vi "TCP Server Lookup Connection Info by Instance VI.vi"(8 "error in (no error)":errorcluster, 10 "Instance VI Refnum":refnum<vi>, 11 "TCP Server":refnum<class "JKI TCP Server.lvclass">) -> (0 "error out":errorcluster, 1 "OK to Start New Handler?":bool, 2 "Connection Info":T2, 3 "TCP Server out":refnum<class "JKI TCP Server.lvclass">, 4 "Additional Data":variant, 5 "Handler VI RefNum":T1)   [LabVIEW 2020, in "JKI TCP Server.lvclass"]
uses:
  JKI TCP Server.lvclass
  _Data Structures/TCP Server Connection Info Cluster.ctl
  _Data Structures/TCP Server Handler RefNum.ctl
  JKI TCP Server.lvclass/JKI TCP Server.ctl
panel:
  # "Copyright © 2004-2008 JKI. All rights reserved.\n\nAuthor: Jim Kring [jim.kring@jameskring.com]\n\nThis library is provided \"AS IS\" ,WITHOUT WARRANTIES OR \nCONDITIONS OF ANY KIND, either express or implied.\n\nJames Kring, Inc. -- http://www.jameskring.com"
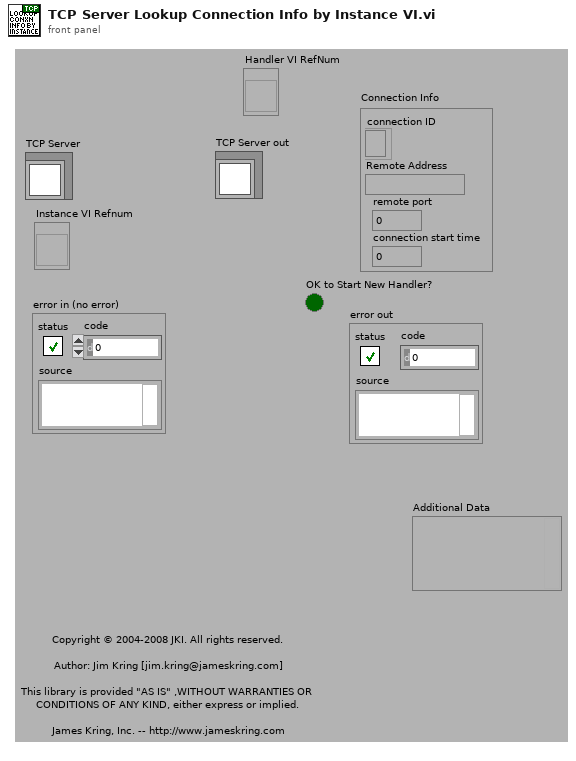
[diagram p1: front panel]
types:
  T1 = typedef "JKI TCP Server.lvclass/TCP Server Handler RefNum.ctl" = refnum<vi>
  T2 = typedef "JKI TCP Server.lvclass/TCP Server Connection Info Cluster.ctl" = cluster{"connection ID":refnum<k5>, "Remote Address":string, "remote port":u16, "connection start time":u32}
  T3 = typedef "JKI TCP Server.lvclass/TCP Server Data.ctl" = cluster{"Listener Info":T4, "Connection Process VI RefNums":refnum<vi>[], "dup connection IDs (for quick search)":refnum<k5>[], "Connections":T2[], "Connection Handler VI Path":path, "Handler Is Reentrant?":bool, "TCP Handler Instance RefNums":T1[], "TCP Handler VI RefNum":T1, "No. Connections":u32, "Max Connections":u32, "server start time":u32, "Additional Data":variant}
  T4 = typedef "JKI TCP Server.lvclass/TCP Server Listener Info Cluster.ctl" = cluster{"listener ID":refnum<k5>, "net address":u32, "port":u16, "Listener Process VI Refnum":refnum<vi>}
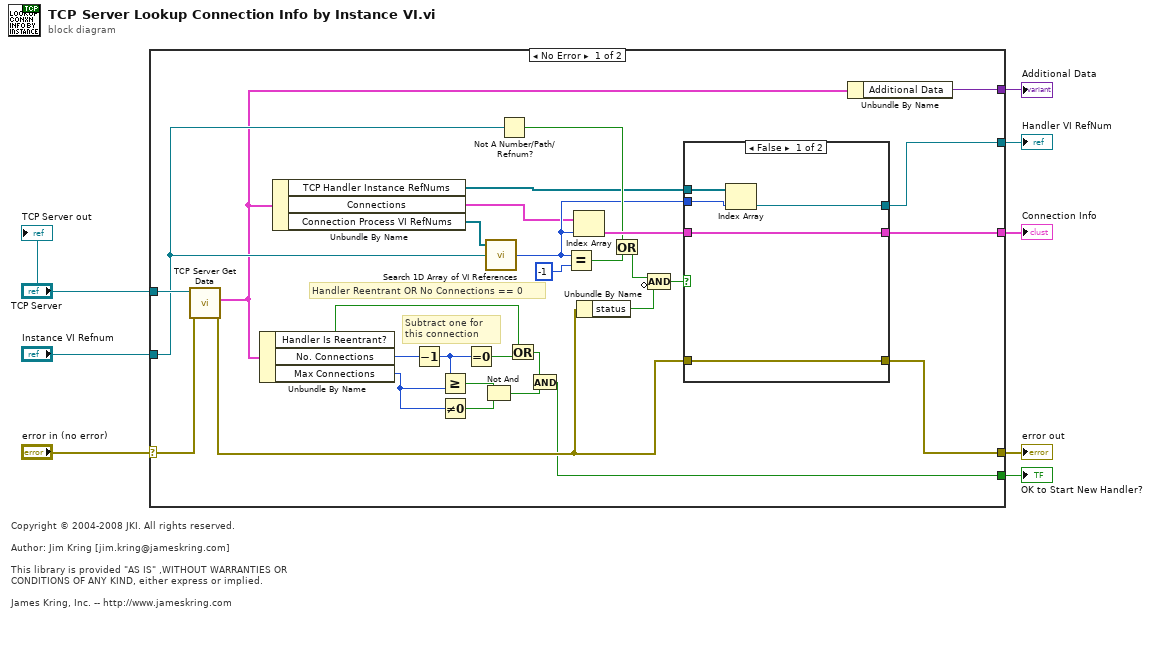
[diagram p0: block diagram]
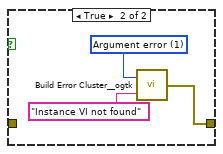
[diagram p2: hidden frame]
diagram:
  # "Copyright © 2004-2008 JKI. All rights reserved.\n\nAuthor: Jim Kring [jim.kring@jameskring.com]\n\nThis library is provided \"AS IS\" ,WITHOUT WARRANTIES OR \nCONDITIONS OF ANY KIND, either express or implied.\n\nJames Kring, Inc. -- http://www.jameskring.com"
  n1 = case shown="No Error" "error in (no error)" {
    tunnel: "TCP Server" -> [w38 _]
    tunnel: "Instance VI Refnum" -> [w27 _]
    tunnel: [w29 w47] -> w7
    selector: "error in (no error)" -> [w36 w47]
    tunnel: [w31 _] -> w4
    tunnel: [w22 _] -> w3
    tunnel: [w13 _] -> w2
    tunnel: [w10 _] -> w1
    frame No Error {
      # "Subtract one for this connection"
      # "Handler Reentrant OR No Connections == 0"
      n2 = call "TCP Server Get Data.vi"("error in (no error)"=w36, "TCP Server"=w38) -> ("error out"=w30:errorcluster, "Data out"=w11:T3)  [unwired: 7 in, 1 out]
      n3 = Unbundle By Name(w11) -> ("Handler Is Reentrant?"=w21:bool, "No. Connections"=w19:u32, "Max Connections"=w18:u32)
      n4 = Unbundle By Name(w11) -> ("TCP Handler Instance RefNums"=w24:T1[], "Connections"=w9:T2[], "Connection Process VI RefNums"=w37:refnum<vi>[])
      n5 = Decrement(x=w19) -> (x-1=w12:u32)
      n6 = Greater Or Equal?(x=w12, y=w18) -> (x >= y?=w17:bool)
      n7 = Not Equal To 0?(x=w18) -> (x != 0?=w16:bool)
      n8 = Equal To 0?(x=w12) -> (x = 0?=w20:bool)
      n9 = Not And(1:w16, 2:w17) -> (0:w15:bool)
      n10 = call "Search 1D Array of VI References.vi"("Instance VI Refnum"=w27, "Connection Process VI RefNums"=w37) -> ("index of element"=w23:i32)  [unwired: 1 in]
      n11 = Not A Number/Path/Refnum?(number/path/refnum=w27) -> (NaN/Path/Refnum?=w26:bool)
      n12 = Or(x=w21, y=w20) -> (x .or. y?=w14:bool)
      n13 = And(x=w14, y=w15) -> (x .and. y?=w13:bool)
      n14 = Equal?(x=w23, y=-1) -> (x = y?=w28:bool)
      n15 = Index Array(array=w9, index=w23) -> (element=w32:T2)
      n16 = Unbundle By Name(w30) -> ("status"=w34:bool)
      n17 = Or(x=w26, y=w28) -> (x .or. y?=w25:bool)
      n18 = Compound Arithmetic op=AND(w25, invert w34) -> (w33:bool)
      n19 = case shown="False" w33 {
        tunnel: w32 -> [w43 _]
        tunnel: [w43 _] -> w31
        tunnel: w30 -> [w42 _]
        tunnel: [w42 w44] -> w29
        tunnel: w24 -> [w41 _]
        tunnel: w23 -> [w40 _]
        tunnel: [w39 _] -> w22
        frame False {
          n20 = Index Array(array=w41, index=w40) -> (element=w39:T1)
        }
        frame True {
          w46 = 1 items=["No error", "Argument error", "Memory is full", "Out of zone", "End of file", "File already open", "Generic file I/O error", "File not found", "File permission error", "Disk is full", "Duplicate path", "Too many files open", "System feature not enabled", "Resource file not found", "Cannot add resource", "Resource not found", "Image not found", "Image memory error", "Pen does not exist", "Config type invalid", "Config token not found", "Config parse error", "Config memory error", "Bad external code format", "Bad external code offset", "External code not present", "Null window", "Destroy window error", "Null menu", "Print aborted", "Bad print record", "Print driver error", "Windows error during printing", "Memory error during printing", "Print dialog error", "Generic print error", "Invalid device refnum", "Device not found", "Device parameter error", "Device unit error", "Cannot open device", "Device call aborted", "Generic error", "Cancelled by user", "Object ID too low", "Object ID too high", "Object not in heap", "Unknown heap", "Unknown object (invalid DefProc)", "Unknown object (DefProc not in table)", "Message out of range", "Invalid (null) method", "Unknown message", "Manager call not supported", "Bad address", "Network operation in progress", "Network operation timed out", "Connection is busy", "Network attribute not supported", "Network error", "Address in use", "System out of memory", "Connection aborted", "Connection refused", "Not connected", "Already connected", "Connection closed", "Initialization error (interapplication manager)", "Bad occurrence", "Wait on unbound occurrence handler", "Occurrence queue overflow", "Datalog type conflict", "Unused", "Unrecognized type (interapplication manager)", "Memory corrupt", "Failed to make temporary DLL", "Old CIN version", "Drag socket not found", "Failed to load drop-object", "Failed to register OLE object", "Failed to release OLE object", "Format specifier type mismatch", "Unknown format specifier", "Too few format specifiers", "Too many format specifiers", "Scan failed", "Newer CIN version", "Error converting to variant", "Runtime menu error", "Password tampered", "Variant attribute not found", "Incompatible variant data type", "Event data is not available", "Event Store is not present", "Occurrence is not found", "Event Queue is not created", "Event info is not available", "Refnum passed is NULL", "Error retrieving Class GUID", "Error retrieving CoClass GUID", "Error retrieving TypeLib GUID.", "Bad built application magic bytes.", "Specific driver is different from the specific driver associated with the Logical Name.", "There is no session opened to the class driver.", "Max Error", "MAX - Error with config objects", "MAX - Error loading configuration", "MAX - Group not supported"]
          n21 = call <userlib>:"Build Error Cluster__ogtk.vi"("String to Prepend to source (\"\")"="Instance VI not found" ("String to Prepend to source (\"\")"), "code"=w46) -> ("error out"=w44:errorcluster)
        }
      }
      n22 = Unbundle By Name(w11) -> ("Additional Data"=w10:variant)
    }
    frame Error {
    }
  }
  "error out" <- w7
  "Connection Info" <- w4
  "Handler VI RefNum" <- w3
  "OK to Start New Handler?" <- w2
  "Additional Data" <- w1
  "TCP Server out" <- "TCP Server"
